vi "HS_Init.vi"(8 "error in":errorcluster, 11 "VISA Refnum in":refnum<visa-resource-name>) -> (0 "error out":errorcluster, 3 "VISA Refnum out":refnum<visa-resource-name>)   [LabVIEW 2017]
uses:
  <vilib>/Instr/_visa.llb/VISA Configure Serial Port (Instr).vi
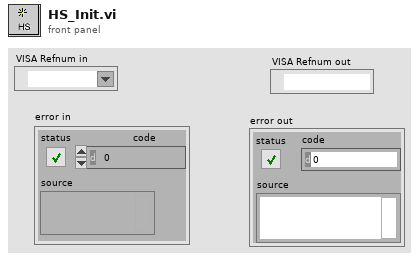
[diagram p1: front panel]
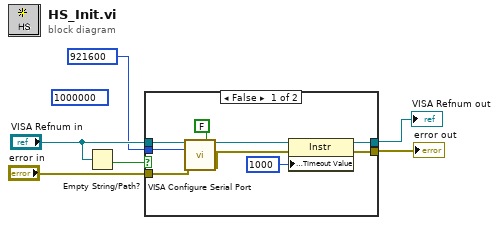
[diagram p0: block diagram]
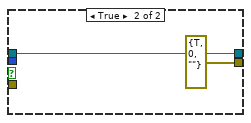
[diagram p2: hidden frame]
diagram:
  (unwired) u32 1000000 ("baud rate (115200)")
  n1 = Empty String/Path?(string/path="VISA Refnum in") -> (empty?=w2:bool)
  n2 = case shown="False" w2 {
    tunnel: [w15 w17] -> w6
    tunnel: "error in" -> [w11 _]
    tunnel: [w9 errorcluster {"status"=TRUE, "code"=0, "source"=""} ("error out")] -> w4
    tunnel: u32 921600 ("baud rate (115200)") -> [w8 _]
    tunnel: "VISA Refnum in" -> [w7 w17]
    frame False {
      n3 = call-poly "VISA Configure Serial Port"("VISA resource name"=w7, "Enable Termination\nChar (T)"=FALSE ("Enable Termination\nChar (T)"), "baud rate (9600)"=w8, "error in (no error)"=w11) -> ("VISA resource name out"=w14:refnum<visa-resource-name>, "error out"=w10:errorcluster)  [unwired: 10 in]
      n4 = property class="Instr"(reference=w14, error in=w10, "General Settings:Timeout Value"=u32 1000) -> (reference out=w15:refnum<visa-resource-name>, error out=w9:errorcluster)
    }
    frame True {
    }
  }
  "VISA Refnum out" <- w6
  "error out" <- w4
